vi "Event Nested.vi"(8 "Alias":string, 10 "Msg":refnum<class "Msg.lvclass">, 11 "Hello World Queue in":refnum<class "Hello World Queue.lvclass">) -> (3 "Hello World Queue out":refnum<class "Hello World Queue.lvclass">)   [LabVIEW 2021, in "Hello World Queue.lvlib" / "Hello World Queue.lvclass"]
uses:
  Hello World Queue.lvclass
  jettl/Msg Strategy/Msg/Msg.lvclass
  Hello World Queue.lvclass/Hello World Queue.ctl
  jettl/jettl/Queue Actor/Queue Actor.lvclass
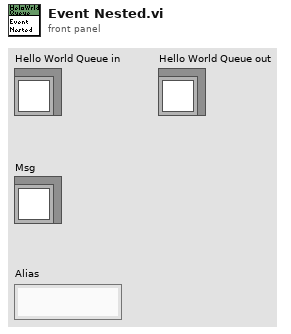
[diagram p1: front panel]
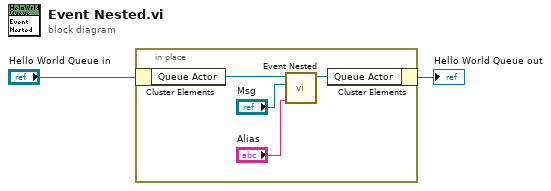
[diagram p0: block diagram]
diagram:
  n1 = in-place {
    n2 = in-place-cluster #1("Hello World Queue in") -> ("Queue Actor"=w6:refnum<class "Queue Actor.lvclass">)
    n3 = call-dynamic "Event Nested.vi"("Alias"="Alias", "Msg"="Msg", "Queue Actor in"=w6) -> ("Queue Actor out"=w5:refnum<class "Queue Actor.lvclass">)  [unwired: 8 in]
    n4 = in-place-cluster #1("Queue Actor"=w5) -> (→"Hello World Queue out":refnum<class "Hello World Queue.lvclass">)
  }
